vi "init-can-frame.vi"(4 "selected.frame":T3={"Comment"="", "Extended Identifier?"=FALSE, "Transmit Time"=0.0, "Timing Type"=1, "Payload Length"=8, "Identifier"=1, "Frame name"="frame1"} {"Timing Type" items=["Cyclic Data", "Event Data", "Cyclic Remote", "Event Remote"]; "Identifier" format="%010x"}) -> (1 "CAN frame":T1 {"payload" format="%x"; "timestamp" format="%<%.7X\n%x>T"; "type" items=["CAN Data"=0, "CAN Remote"=1, "CAN Bus Error"=2, "J1939 Data"=192, "Delay"=224, "Log Trigger"=225, "Start Trigger"=226]; "identifier" format="%x"}, 2 "Identifier":u32)   [LabVIEW 2015]
uses:
  class.dbc/controls/dbc-frame.ctl
  <vilib>/xnet/xnet.llb/XNET Frame CAN.ctl
  <vilib>/xnet/xnet.llb/XNET Frame Type CAN.ctl
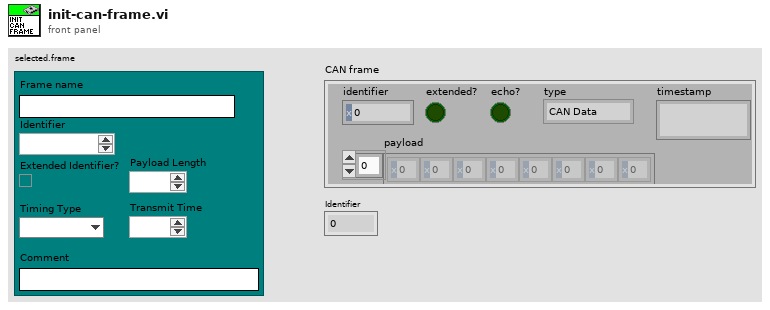
[diagram p1: front panel]
types:
  T1 = typedef "XNET Frame CAN.ctl" = cluster{"timestamp":timestamp, "payload":u8[], "identifier":u32, "type":T2, "extended?":bool, "echo?":bool}
  T2 = typedef "XNET Frame Type CAN.ctl" = u8
  T3 = typedef "dbc-frame.ctl" = cluster{"Comment":string, "Extended Identifier?":bool, "Transmit Time":dbl, "Timing Type":u32, "Payload Length":u32, "Identifier":u32, "Frame name":string}
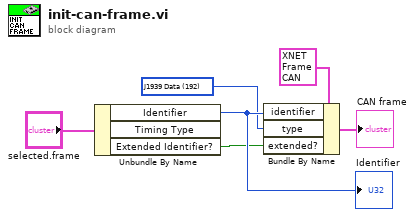
[diagram p0: block diagram]
diagram:
  w1 = T2 192 items=["CAN Data"=0, "CAN Remote"=1, "CAN Bus Error"=2, "J1939 Data"=192, "Delay"=224, "Log Trigger"=225, "Start Trigger"=226] ("type")
  n1 = Unbundle By Name("selected.frame") -> ("Identifier"=w3:u32, "Extended Identifier?"=w2:bool)  [unwired: 1 out]
  "Identifier" <- w3
  n2 = Bundle By Name(cluster=T1 {"timestamp"=timestamp(0 s since 1904-01-01), "payload"=[], "identifier"=0, "type"=0, "extended?"=FALSE, "echo?"=FALSE} ("CAN frame"), "identifier"=w3, "type"=w1, "extended?"=w2) -> (→"CAN frame":T1)
